vi "setup_lc_tc.vi"(0 "didian":string, 4 "shuoming":string, 6 "jsren":string, 9 "yw":string, 10 "id":string, 11 "zc_luodi_num":string) -> (2 "error":errorcluster caption="error out 2")   [LabVIEW 2017, in "Lib_code.lvlib"]
uses:
  Lib_code.lvlib
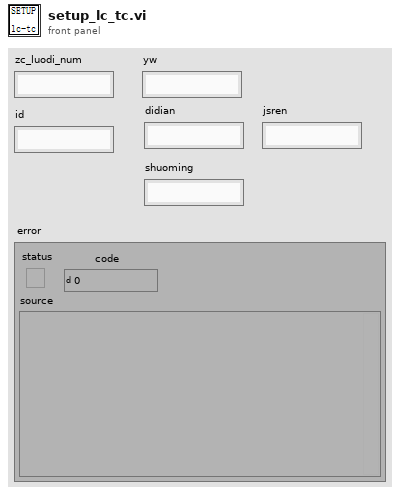
[diagram p1: front panel]
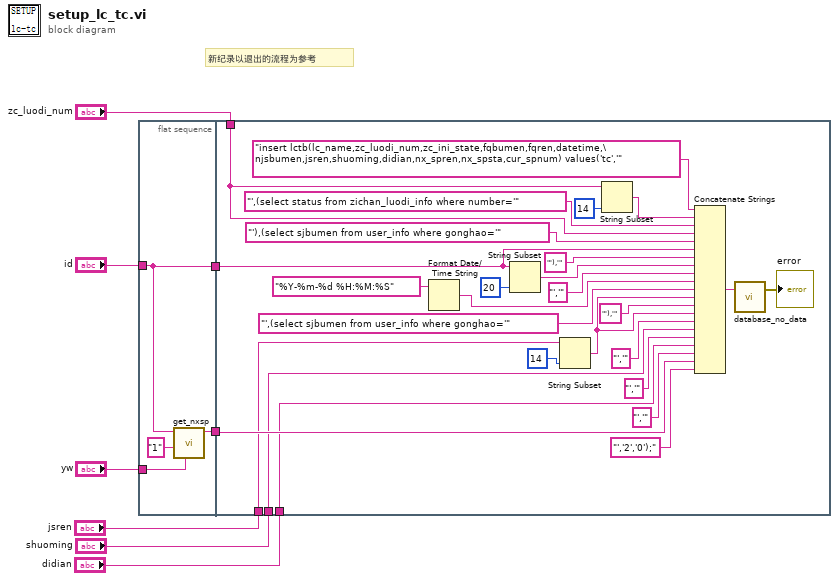
[diagram p0: block diagram]
diagram:
  # "新纪录以退出的流程为参考"
  n1 = flat-sequence {
    tunnel: "id" -> [w11]
    tunnel: [w11] -> w7
    tunnel: [w12] -> w6
    tunnel: "yw" -> [w10]
    tunnel: w7 -> [w28]
    tunnel: w6 -> [w27]
    tunnel: "zc_luodi_num" -> [w24]
    tunnel: "shuoming" -> [w17]
    tunnel: "didian" -> [w19]
    tunnel: "jsren" -> [w15]
    frame #0 {
      n2 = call "get_nxsp.vi"("yw"=w10, "Cur_state"="1", "fqren"=w11) -> ("sp_gonghao"=w12:string)  [unwired: 6 in, 2 out]
    }
    frame #1 {
      n3 = Format Date/Time String(time format string (%c)="%Y-%m-%d %H:%M:%S" ("时间格式字符串(%c)")) -> (date/time string=w29:string)  [unwired: 2 in]
      n4 = String Subset(string=w28, length (rest)=20 ("长度（剩余）")) -> (substring=w31:string)  [unwired: 1 in]
      n5 = String Subset(string=w15, length (rest)=14 ("长度（剩余）")) -> (substring=w13:string)  [unwired: 1 in]
      n6 = String Subset(string=w24, length (rest)=14 ("长度（剩余）")) -> (substring=w37:string)  [unwired: 1 in]
      n7 = Concatenate Strings("insert lctb(lc_name,zc_luodi_num,zc_ini_state,fqbumen,fqren,datetime,\njsbumen,jsren,shuoming,didian,nx_spren,nx_spsta,cur_spnum) values('tc','" ("格式字符串"), w37, "',(select status from zichan_luodi_info where number='" ("字符串"), w24, "'),(select sjbumen from user_info where gonghao='" ("字符串"), w28, "'),'" ("字符串"), w31, "','" ("字符串"), w29, "',(select sjbumen from user_info where gonghao='" ("字符串"), w13, "'),'" ("字符串"), w13, "','" ("字符串"), w17, "','" ("字符串"), w19, "','" ("字符串"), w27, "','2','0');" ("字符串")) -> (w22:string)
      n8 = call "database_no_data.vi"("input"=w22) -> ("error"=→"error":errorcluster)  [unwired: 2 in]
    }
  }
